vi "example_microFPGA_PWM.vi"() -> ()   [LabVIEW 2021]
panel:
  out "PWM_ratio_READ":u32(slide)=49 max=255 step=1 scale=0.0..255.0 scale format="%u us"
  in  "PWM_channel":u16(ring)=3 items=["channel No 0", "channel No 1", "channel No 2", "channel No 3", "channel No 4"]
  in  "write or read":u16(ring)=1 items=["read", "write"]
  out "value write confirm 4":bool
  out "Version":u16=3
  in  "PWM ratio":u32(slide)=49 max=255 step=1 scale=0.0..255.0 scale format="%u us"
  in  "close Application":bool=TRUE
  in  "send parameters":bool
  # "PWM control"
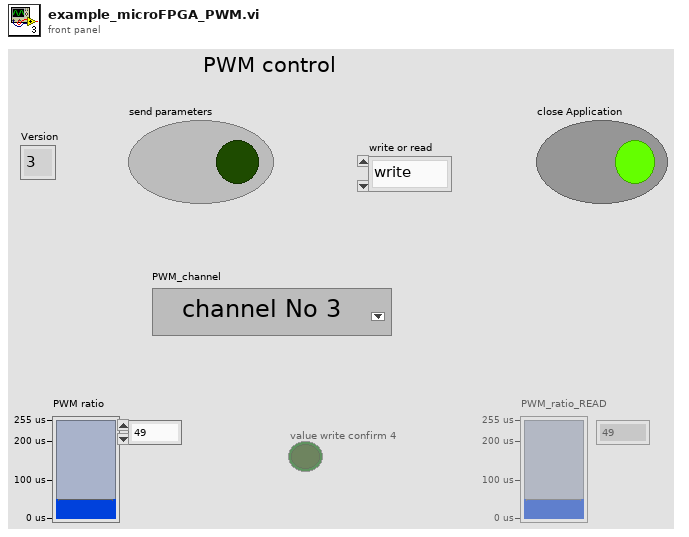
[diagram p1: front panel]
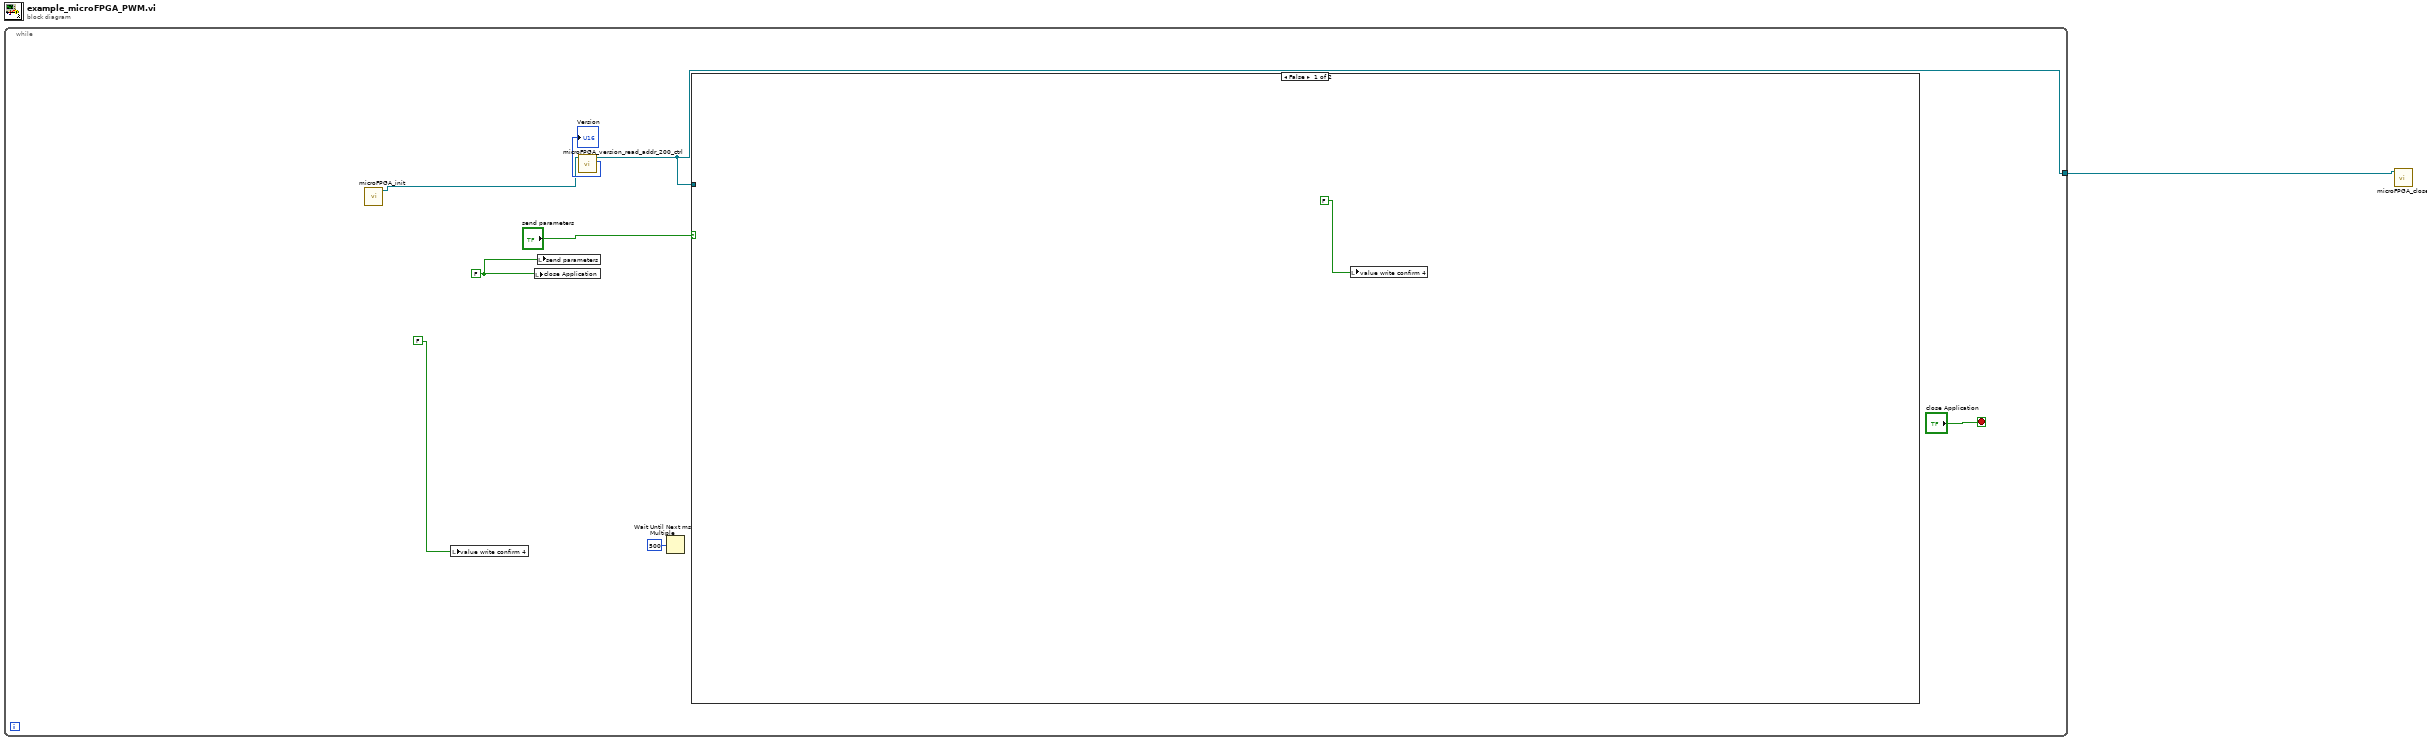
[diagram p0: block diagram]
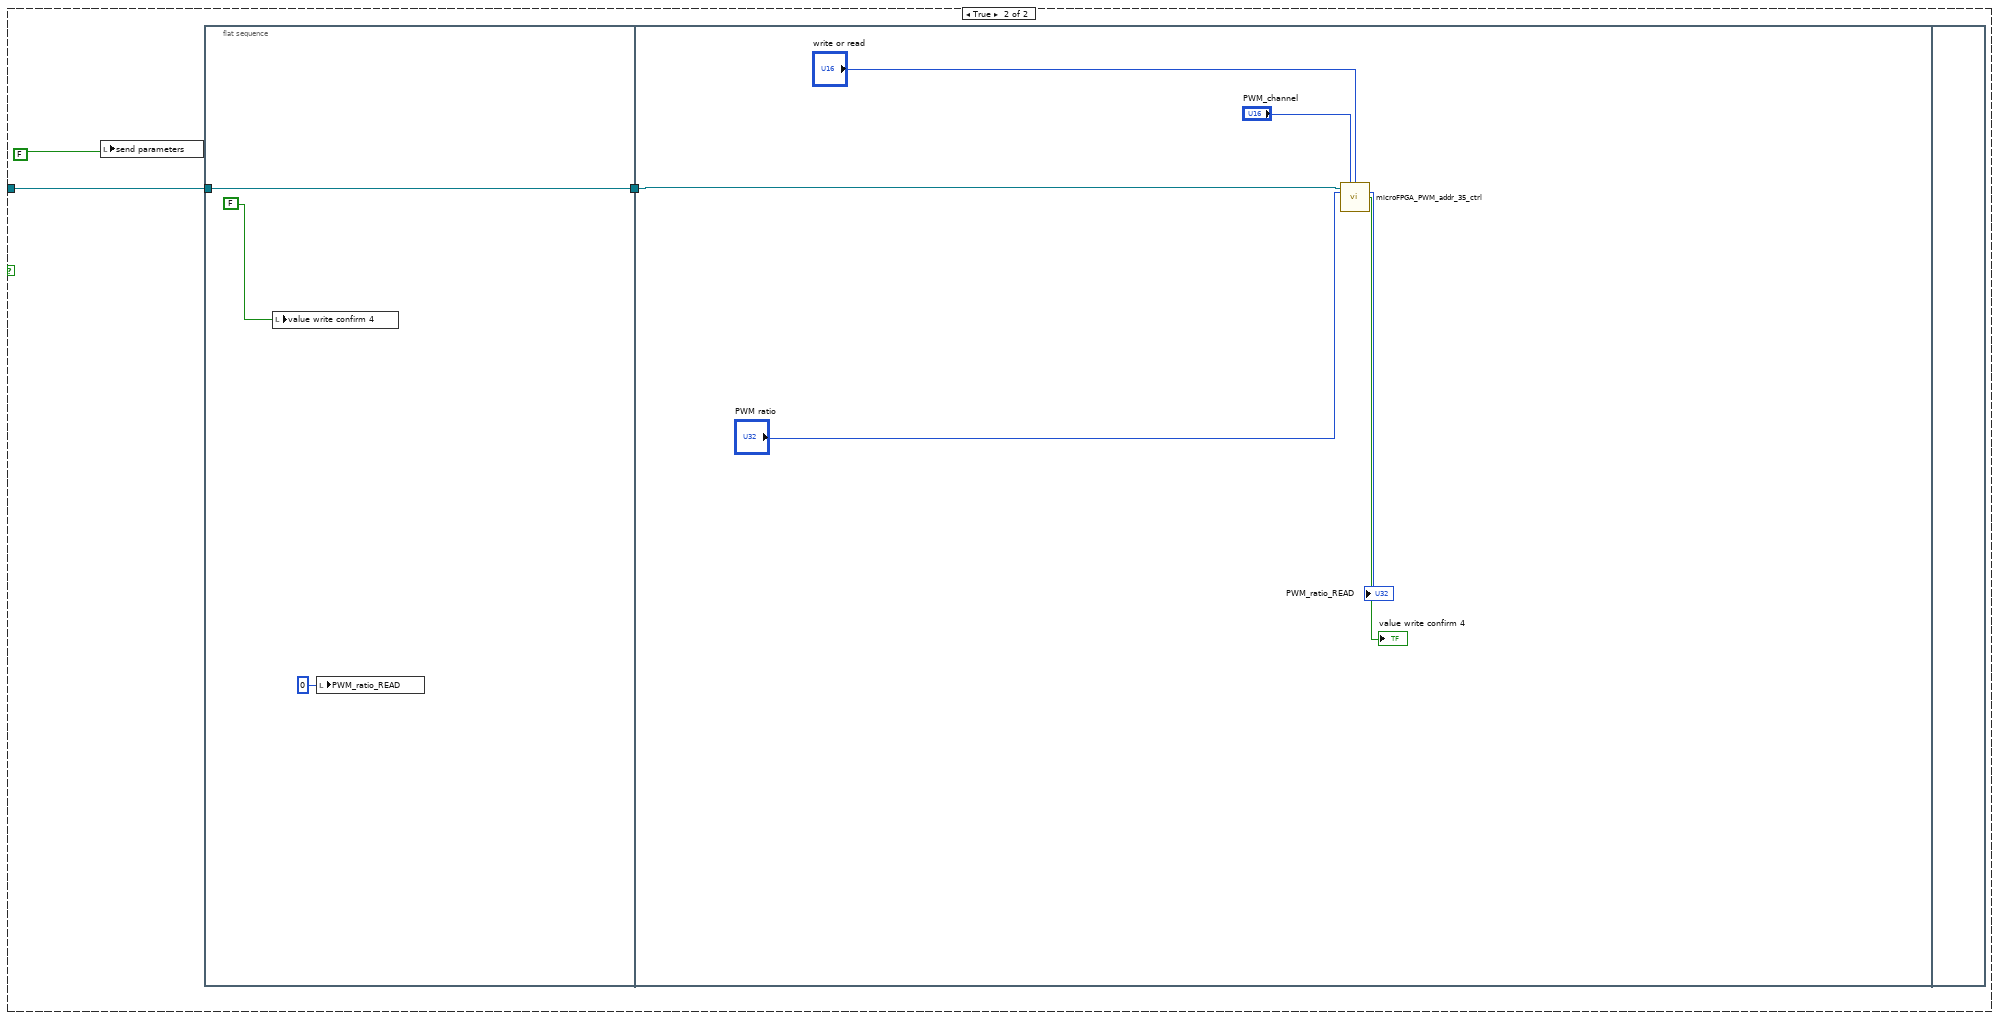
[diagram p2: hidden frame]
diagram:
  n1 = while {
    tunnel: [w5] -> w1
    stop <- "close Application" stop-if-true
    w2 = FALSE ("write")
    n2 = call "microFPGA_init.vi"() -> ("VISA resource name out"=w3:refnum<visa-resource-name>)  [unwired: 10 in, 1 out]
    n3 = local write "value write confirm 4"(FALSE ("write")) -> ()
    n4 = local write "close Application"(w2) -> ()
    n5 = local write "send parameters"(w2) -> ()
    n6 = call "microFPGA_version_read_addr_200_ctrl.vi"("VISA resource name"=w3) -> ("VISA resource name 2"=w5:refnum<visa-resource-name>, "Version"=→"Version":u16)  [unwired: 12 in, 1 out]
    n7 = Wait Until Next ms Multiple(millisecond multiple=u32 500) -> ()  [unwired: 1 out]
    n8 = case shown="False" "send parameters" {
      tunnel: w5 -> [_ w12]
      frame False {
        n9 = local write "value write confirm 4"(FALSE ("value write confirm")) -> ()
      }
      frame True {
        n10 = local write "send parameters"(FALSE ("write")) -> ()
        n11 = flat-sequence {
          tunnel: w12 -> [w16]
          tunnel: [w16] -> w11
          tunnel: w11 -> [w17]
          frame #0 {
            n12 = local write "value write confirm 4"(FALSE ("value write confirm")) -> ()
            n13 = local write "PWM_ratio_READ"(u32 0 ("PWM_ratio_READ")) -> ()
          }
          frame #1 {
            n14 = call "microFPGA_PWM_addr_35_ctrl.vi"("VISA resource name"=w17, "PWM_channel"="PWM_channel", "write or read"="write or read", "PWM_ratio_WRITE"="PWM ratio") -> ("PWM_ratio_READ"=→"PWM_ratio_READ":u32, "value write confirm"=→"value write confirm 4":bool)  [unwired: 7 in, 3 out]
          }
          frame #2 {
          }
        }
      }
    }
  }
  n15 = call "microFPGA_close.vi"("VISA resource name"=w1) -> ()  [unwired: 11 in]
